vi "extract single slice img from a frame (SubVI).vi"(8 "AOD scan speed ratio":dbl, 9 "init pos":dbl, 10 "Nx":dbl, 11 "image in":u16[][](array[numeric])) -> (3 "Array":u16[][](array[numeric]))   [LabVIEW 2024]
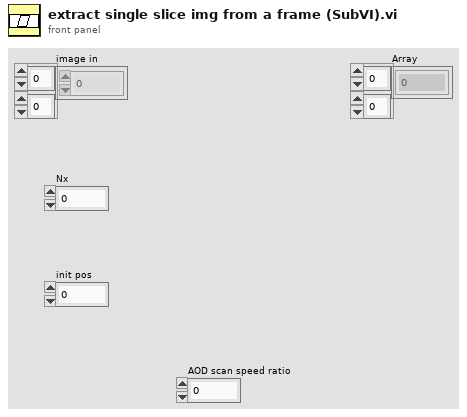
[diagram p1: front panel]
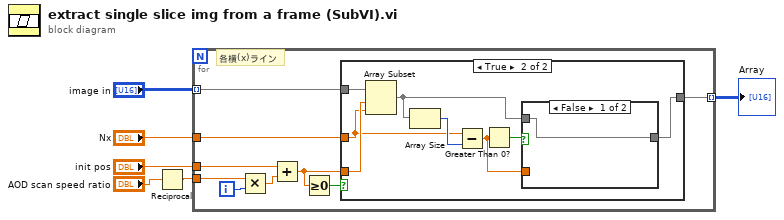
[diagram p0: block diagram]
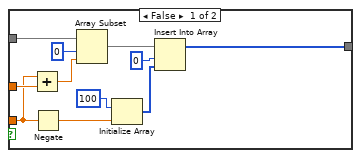
[diagram p2: hidden frame]
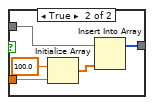
[diagram p3: hidden frame]
diagram:
  n1 = Reciprocal(x="AOD scan speed ratio") -> (1/x=w1:dbl)
  n2 = for {
    tunnel: "image in" -> [w15] mode=indexing
    tunnel: "init pos" -> [w14]
    tunnel: w1 -> [w11]
    tunnel: [w10] -> w6 mode=indexing
    tunnel: "Nx" -> [w8]
    i -> [w13]
    # "各横(x)ライン"
    n3 = Multiply(x=w11, y=w13) -> (x*y=w12:dbl)
    n4 = Add(x=w14, y=w12) -> (x+y=w9:dbl)
    n5 = Greater Or Equal To 0?(x=w9) -> (x >= 0?=w7:bool)
    n6 = case shown="True" w7 {
      tunnel: w15 -> [w26 w34]
      tunnel: [w16 w27] -> w10
      tunnel: w9 -> [w22 w33]
      tunnel: w8 -> [w24 w31]
      frame False {
        n7 = Add(x=w22, y=w24) -> (x+y=w23:dbl)
        n8 = Negate(x=w22) -> (-x=w21:dbl)
        n9 = Array Subset(array=w26, index=0, length=w23) -> (w17:u16[])
        n10 = Initialize Array(u16 100 ("element"), w21) -> (w19:u16[])
        n11 = Insert Into Array(array=w17, index=0, new element=w19) -> (w16:u16[])
      }
      frame True {
        n12 = Array Subset(array=w34, index=w33, length=w31) -> (w29:u16[])
        n13 = Array Size(array=w29) -> (size(s)=w32:i32)
        n14 = Subtract(x=w31, y=w32) -> (x-y=w28:dbl)
        n15 = Greater Than 0?(x=w28) -> (x > 0?=w30:bool)
        n16 = case shown="False" w30 {
          tunnel: w29 -> [w35 w40]
          tunnel: w28 -> [_ w39]
          tunnel: [w35 w36] -> w27
          frame False {
          }
          frame True {
            n17 = Initialize Array(100.0 ("element"), w39) -> (w37:dbl[])
            n18 = Insert Into Array(array=w40, new element=w37) -> (w36:u16[])  [unwired: 1 in]
          }
        }
      }
    }
  }
  "Array" <- w6
